vi "CRYTS Step Move Down.vi"(11 "Sequence":refnum<vi>) -> ()   [LabVIEW 2013]
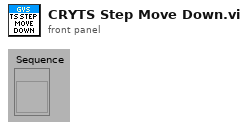
[diagram p1: front panel]
types:
  T1 = enum16{"Insert", "Remove", "Move up", "Move down"}
  T2 = cluster{"SourceRowNum":i32, "SourceCount":i32, "TargetRowNum":i32, "bResult":bool, "EditRowNum":i32}
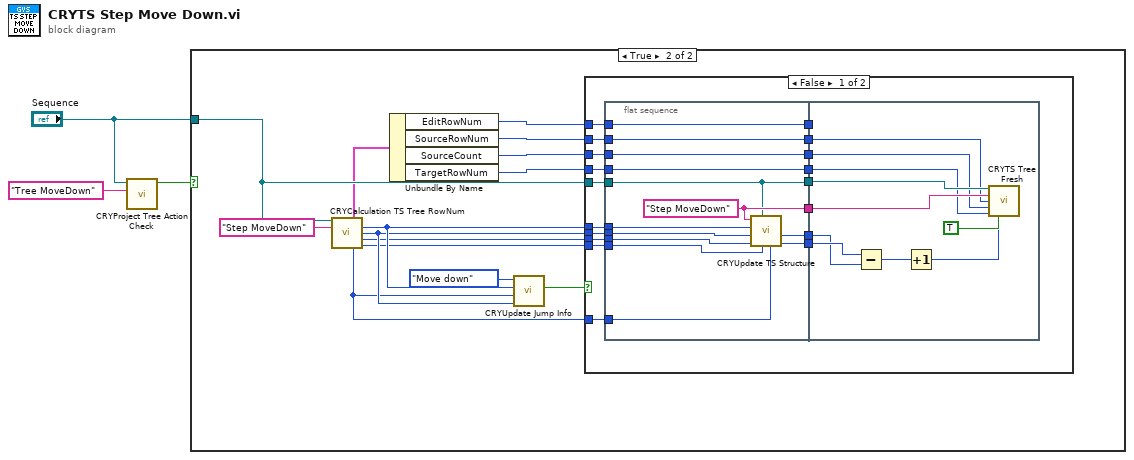
[diagram p0: block diagram]
diagram:
  n1 = call "CRYProject Tree Action Check.vi"("sOption"="Tree MoveDown", "Project Tree reference"="Sequence") -> ("bResult"=w2:bool)  [unwired: 8 in, 1 out]
  n2 = case shown="True" w2 {
    tunnel: "Sequence" -> [_ w16]
    frame False {
    }
    frame True {
      n3 = call "CRYCalculation TS Tree RowNum.vi"("Tree Task SequenceIn"=w16, "sOption"="Step MoveDown") -> ("DispInfo Cluster Out"=w9:T2, "SourceRowNum"=w14:i32, "SourceCount"=w13:i32, "TargetRowNum"=w12:i32, "MoveCount"=w4:i32, "EditRowNum"=w11:i32)  [unwired: 7 in, 1 out]
      n4 = Unbundle By Name(w9) -> ("EditRowNum"=w5:i32, "SourceRowNum"=w8:i32, "SourceCount"=w7:i32, "TargetRowNum"=w6:i32)
      n5 = call "CRYUpdate Jump Info.vi"("SourceCount"=w13, "MoveCount"=w4, "Step number Selected"=w14, "Action"=T1."Move down") -> ("Canceled?"=w10:bool)  [unwired: 6 in, 1 out]
      n6 = case shown="False" w10 {
        tunnel: w16 -> [w34 _]
        tunnel: w14 -> [w33 _]
        tunnel: w13 -> [w32 _]
        tunnel: w12 -> [w31 _]
        tunnel: w11 -> [w30 _]
        tunnel: w8 -> [w27 _]
        tunnel: w7 -> [w25 _]
        tunnel: w6 -> [w23 _]
        tunnel: w5 -> [w21 _]
        tunnel: w4 -> [w18 _]
        frame False {
          n7 = flat-sequence {
            tunnel: [w37] -> w35
            tunnel: [w45] -> w29
            tunnel: [w43] -> w28
            tunnel: [w42] -> w26
            tunnel: [w41] -> w24
            tunnel: [w40] -> w22
            tunnel: [w39] -> w20
            tunnel: [w38] -> w19
            tunnel: w34 -> [w37]
            tunnel: w33 -> [w44]
            tunnel: w32 -> [w38]
            tunnel: w31 -> [w39]
            tunnel: w30 -> [w46]
            tunnel: w27 -> [w43]
            tunnel: w25 -> [w42]
            tunnel: w23 -> [w41]
            tunnel: w21 -> [w40]
            tunnel: w18 -> [w36]
            tunnel: w35 -> [w55]
            tunnel: w29 -> [w54]
            tunnel: w28 -> [w53]
            tunnel: w26 -> [w52]
            tunnel: w24 -> [w51]
            tunnel: w22 -> [_]
            tunnel: w20 -> [w50]
            tunnel: w19 -> [w49]
            frame #0 {
              w45 = "Step MoveDown" ("sOption")
              n8 = call "CRYUpdate TS Structure.vi"("Move Count"=w36, "Edit Step Num"=w46, "Tree Task SequenceIn"=w37, "Target Index"=w39, "Count"=w38, "Source Index"=w44, "sOption"=w45) -> ()  [unwired: 5 in]
            }
            frame #1 {
              n9 = Subtract(x=w50, y=w49) -> (x-y=w48:i32)
              n10 = Increment(x=w48) -> (x+1=w47:i32)
              n11 = call "CRYTS Tree Fresh.vi"("SequenceTree"=w55, "Edit Index"=w47, "sOption"=w54, "Source Index"=w53, "SourceCount"=w52, "Target Index"=w51, "Is Refresh?"=TRUE) -> ()  [unwired: 8 in, 1 out]
            }
          }
        }
        frame True {
        }
      }
    }
  }
